vi "Serial Plotter 5 Values.vi"() -> ()   [LabVIEW 2014]
uses:
  <vilib>/Instr/_visa.llb/VISA Configure Serial Port (Instr).vi
panel:
  out "Transistor Transfer Characteristic":cluster{dbl[], dbl[]}(graph)
  out "String":string="835,951\r\n"
  out "error IO":errorcluster
  in  "baud rate":u32=115200
  out "Arduino measured voltages":cluster{dbl, dbl, dbl, dbl, dbl}(graph)
  in  "stop":bool
  in  "COM port":refnum<visa-resource-name>="COM5"
  in  "error in":errorcluster
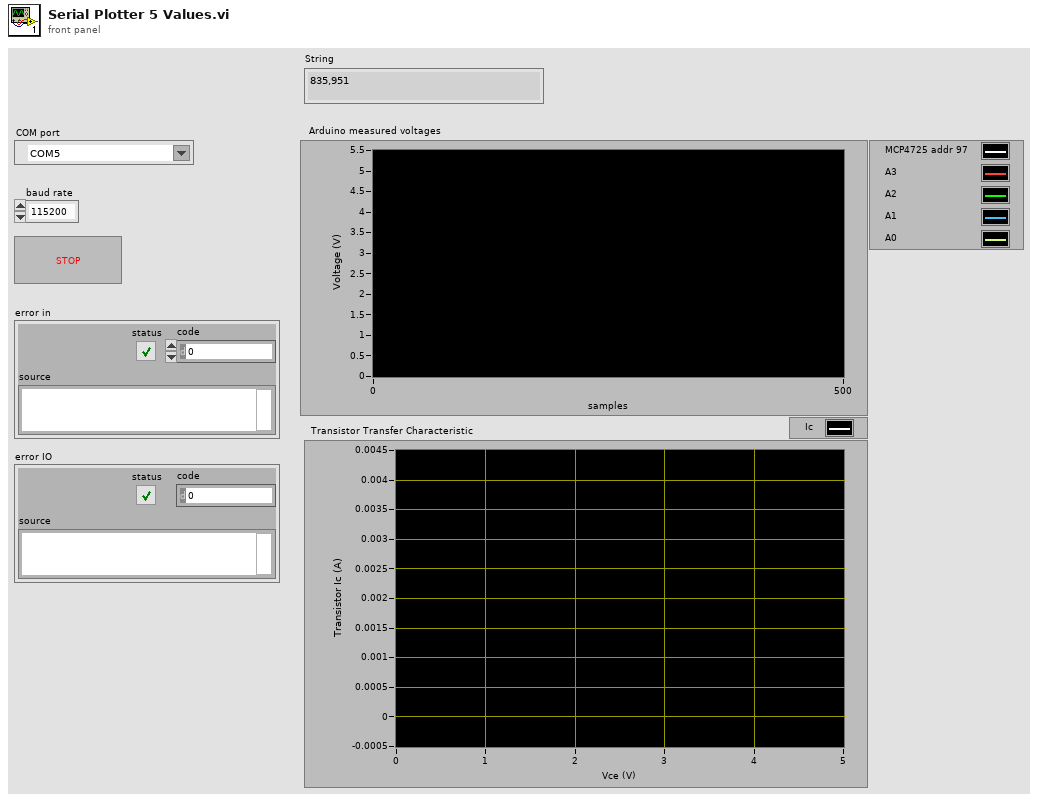
[diagram p1: front panel]
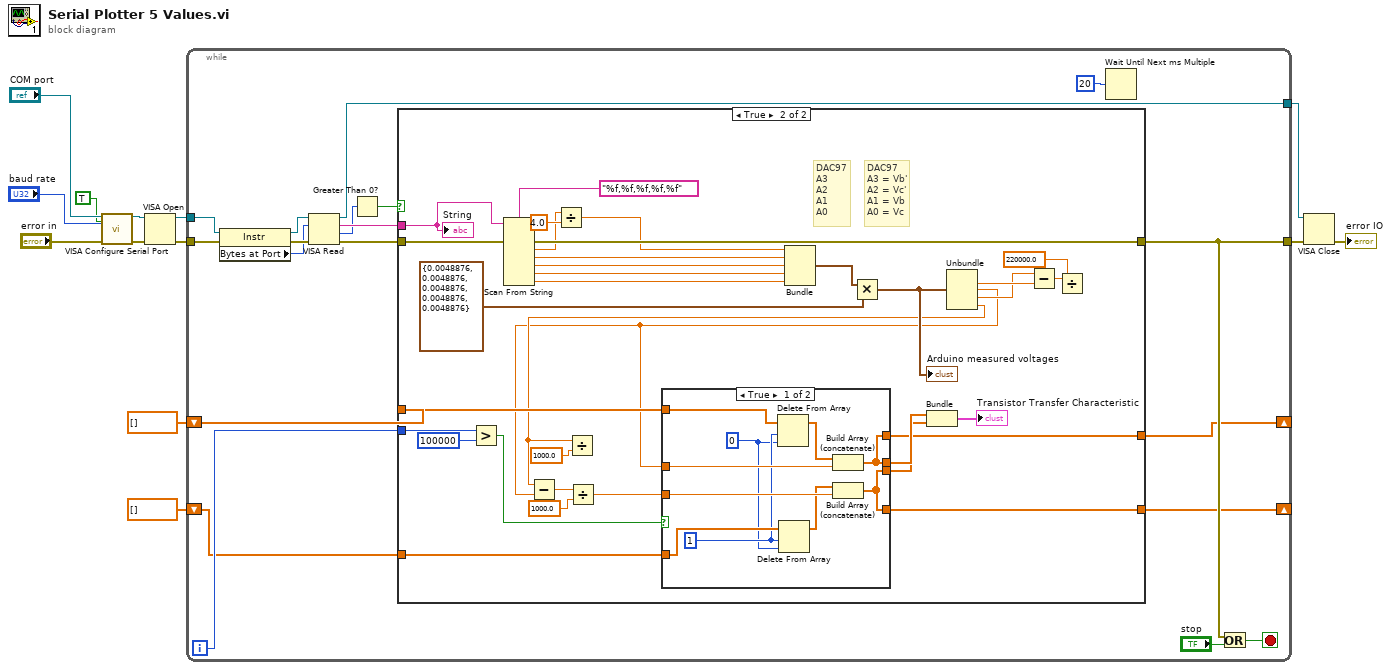
[diagram p0: block diagram]
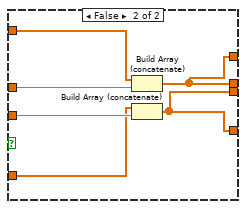
[diagram p3: hidden frame]
diagram:
  n1 = call-poly "VISA Configure Serial Port"("VISA resource name"="COM port", "Enable Termination\nChar (T)"=TRUE ("Enable Termination\nChar (T)"), "baud rate (9600)"="baud rate", "error in (no error)"="error in") -> ("VISA resource name out"=w8:refnum<visa-resource-name>, "error out"=w10:errorcluster)  [unwired: 10 in]
  n2 = VISA Open(error in (no error)=w10, VISA resource name=w8) -> (VISA resource name=w12:refnum<visa-resource-name>, error out=w13:errorcluster)  [unwired: 3 in]
  n3 = while {
    tunnel: w13 -> [w28]
    tunnel: [w22] -> w5
    tunnel: w12 -> [w25]
    tunnel: [w19] -> w3
    shift-right: [w16] -> _
    shift-left: dbl[] [] -> [w17]
    shift-right: [w14] -> _
    shift-left: dbl[] [] -> [w15]
    i -> [w18]
    stop <- w20 stop-if-true
    n4 = property class="Instr"(reference=w25, error in=w28) -> (reference out=w26:refnum<visa-resource-name>, error out=w27:errorcluster, "Bytes at Port"=w24:u32)
    n5 = VISA Read(VISA resource name=w26, byte count=w24, error in (no error)=w27) -> (VISA resource name out=w19:refnum<visa-resource-name>, read buffer=w32:string, return count=w29:u32, error out=w31:errorcluster)
    n6 = Greater Than 0?(x=w29) -> (x > 0?=w30:bool)
    n7 = case shown="True" w30 {
      tunnel: w32 -> [_ w66]
      tunnel: w31 -> [w35 w68]
      tunnel: [w35 w67] -> w22
      tunnel: w18 -> [_ w62]
      tunnel: w17 -> [w34 w59]
      tunnel: [w34 w58] -> w16
      tunnel: w15 -> [w33 w57]
      tunnel: [w33 w56] -> w14
      frame False {
      }
      frame True {
        # "DAC97\nA3 = Vb'\nA2 = Vc'\nA1 = Vb\nA0 = Vc"
        # "DAC97\nA3\nA2\nA1\nA0"
        n8 = Greater?(x=w62, y=100000) -> (0:w60:bool)
        n9 = Scan From String(format string="%f,%f,%f,%f,%f", input string=w66, error in=w68) -> (error out=w67:errorcluster, output 1=w53:dbl, output 2=w50:dbl, output 3=w44:dbl, output 4=w55:dbl, output 5=w45:dbl)  [unwired: 6 in, 2 out]
        n10 = Divide(x=w53, y=4.0) -> (x/y=w46:dbl)
        n11 = Bundle(w46, w50, w44, w55, w45) -> (w51:cluster{dbl, dbl, dbl, dbl, dbl})  [unwired: 1 in]
        n12 = Multiply(x=w51, y=cluster{dbl, dbl, dbl, dbl, dbl} {0.0048876, 0.0048876, 0.0048876, 0.0048876, 0.0048876}) -> (x*y=w47:cluster{dbl, dbl, dbl, dbl, dbl})
        "Arduino measured voltages" <- w47
        n13 = Unbundle(w47) -> (w41:dbl, w36:dbl, w39:dbl, w37:dbl)  [unwired: 1 out]
        n14 = Subtract(x=w37, y=w36) -> (x-y=w49:dbl)
        n15 = Divide(x=w37, y=1000.0) -> ()  [unwired: 1 out]
        n16 = Divide(x=w49, y=1000.0) -> (x/y=w38:dbl)
        n17 = case shown="True" w60 {
          tunnel: w36 -> [w79 w85]
          tunnel: w38 -> [w78 w84]
          tunnel: [w75 w82] -> w64
          tunnel: [w73 w80] -> w63
          tunnel: w59 -> [w72 w83]
          tunnel: [w75 w82] -> w58
          tunnel: w57 -> [w74 w81]
          tunnel: [w73 w80] -> w56
          frame True {
            w70 = 0 ("index")
            w71 = 1 ("index")
            n18 = Delete From Array(array=w72, length=w71, index=w70) -> (array with subset deleted=w77:dbl[])  [unwired: 1 out]
            n19 = Delete From Array(array=w74, length=w71, index=w70) -> (array with subset deleted=w76:dbl[])  [unwired: 1 out]
            n20 = Build Array (concatenate)(w77, w79) -> (w75:dbl[])
            n21 = Build Array (concatenate)(w76, w78) -> (w73:dbl[])
          }
          frame False {
            n22 = Build Array (concatenate)(w83, w85) -> (w82:dbl[])
            n23 = Build Array (concatenate)(w81, w84) -> (w80:dbl[])
          }
        }
        n24 = Bundle(w64, w63) -> (→"Transistor Transfer Characteristic":cluster{dbl[], dbl[]})  [unwired: 1 in]
        n25 = Subtract(x=w39, y=w41) -> (x-y=w43:dbl)
        n26 = Divide(x=w43, y=220000.0) -> ()  [unwired: 1 out]
        "String" <- w66
      }
    }
    n27 = Wait Until Next ms Multiple(millisecond multiple=u32 20) -> ()  [unwired: 1 out]
    n28 = Or(x=w22, y="stop") -> (x .or. y?=w20:bool)
  }
  n29 = VISA Close(VISA resource name=w3, error in (no error)=w5) -> (error out=→"error IO":errorcluster)
